vi "Transfer_U16_IMG_to_Str.vi"(1 "[IN] U16 Pixel Img":u16[][](array[numeric])) -> (0 "[OUT] Converted String":string)   [LabVIEW 2020]
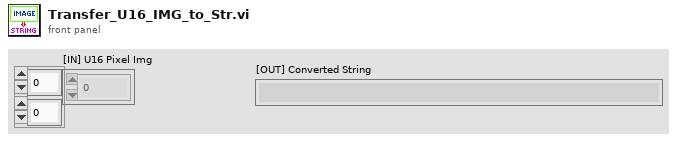
[diagram p1: front panel]
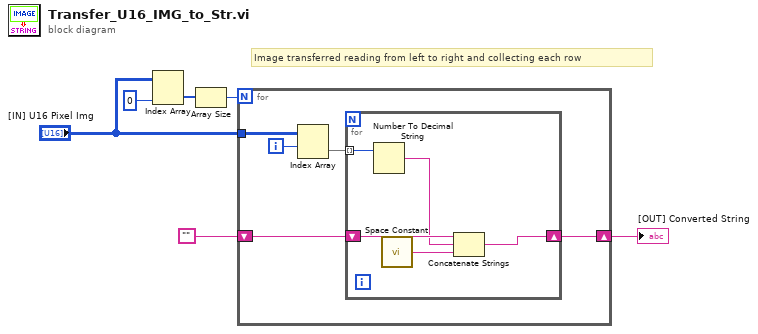
[diagram p0: block diagram]
diagram:
  # "Image transferred reading from left to right and collecting each row"
  n1 = Index Array(array="[IN] U16 Pixel Img", index (col)=0 ("disabled index (col)")) -> (element=w5:u16[])  [unwired: 1 in]
  n2 = Array Size(array=w5) -> (size(s)=w4:i32)
  n3 = for {
    N: w4 -> [_]
    tunnel: "[IN] U16 Pixel Img" -> [w11]
    shift-right: [w7] -> w1
    shift-left: "" -> [w8]
    i -> [w10]
    n4 = Index Array(array=w11, index (row)=w10) -> (element=w9:u16[])  [unwired: 1 in]
    n5 = for {
      tunnel: w9 -> [w16] mode=indexing
      shift-right: [w12] -> w7
      shift-left: w8 -> [w15]
      n6 = Number To Decimal String(number=w16) -> (decimal integer string=w14:string)  [unwired: 1 in]
      n7 = call <vilib>:"Space Constant.vi"() -> ("String"=w13:string)
      n8 = Concatenate Strings(w15, w14, w13) -> (w12:string)
    }
  }
  "[OUT] Converted String" <- w1
